vi "IP Address - Get.vi"(11 "error in (no error)":errorcluster) -> (4 "return code":i32, 6 "LAN IP Address":string, 8 "LAN Subnet Mask":string, 15 "error out":errorcluster)   [LabVIEW 2009]
panel:
  out "Wireless IP Address":string
  out "Wireless Subnet Mask":string
  out "standard output":string
  out "standard error":string
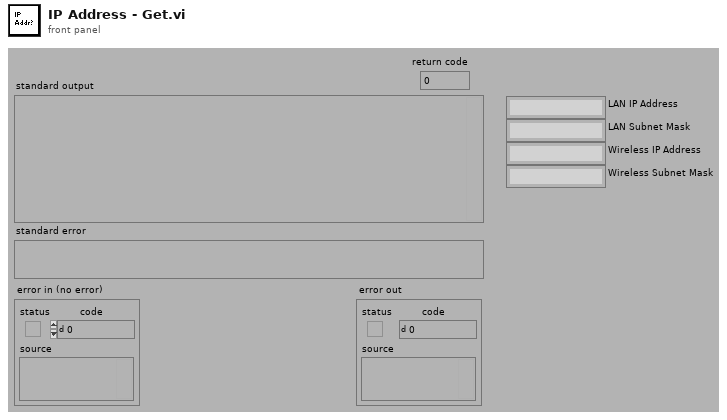
[diagram p1: front panel]
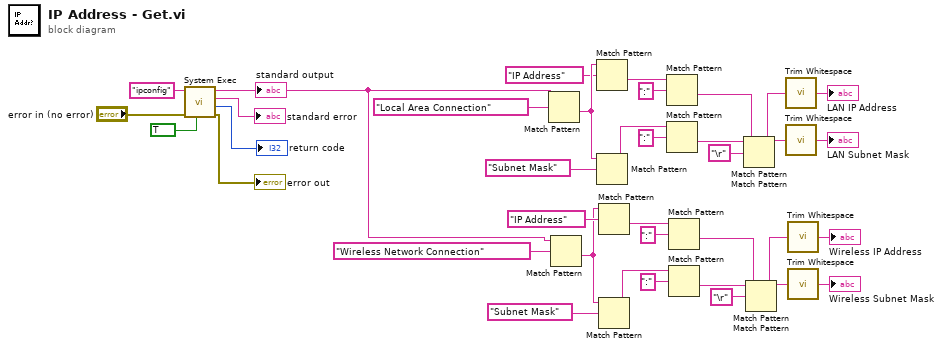
[diagram p0: block diagram]
diagram:
  n1 = call <vilib>:"System Exec.vi"("run minimized? (F)"=TRUE, "error in (no error)"="error in (no error)", "command line"="ipconfig") -> ("error out"=→"error out":errorcluster, "return code"=→"return code":i32, "standard error"=→"standard error":string, "standard output"=w1:string)  [unwired: 5 in]
  "standard output" <- w1
  n2 = Match Pattern(string=w1, regular expression="Local Area Connection" ("command line")) -> (after substring=w27:string)  [unwired: 1 in, 3 out]
  n3 = Match Pattern(string=w1, regular expression="Wireless Network Connection" ("command line")) -> (after substring=w11:string)  [unwired: 1 in, 3 out]
  n4 = Match Pattern(string=w27, regular expression="IP Address" ("command line")) -> (after substring=w35:string)  [unwired: 1 in, 3 out]
  n5 = Match Pattern(string=w27, regular expression="Subnet Mask" ("command line")) -> (after substring=w30:string)  [unwired: 1 in, 3 out]
  n6 = Match Pattern(string=w11, regular expression="IP Address" ("command line")) -> (after substring=w3:string)  [unwired: 1 in, 3 out]
  n7 = Match Pattern(string=w11, regular expression="Subnet Mask" ("command line")) -> (after substring=w8:string)  [unwired: 1 in, 3 out]
  n8 = Match Pattern(string=w35, regular expression=":" ("command line")) -> (after substring=w28:string)  [unwired: 1 in, 3 out]
  n9 = Match Pattern(string=w30, regular expression=":" ("command line")) -> (after substring=w29:string)  [unwired: 1 in, 3 out]
  n10 = Match Pattern(string=w3, regular expression=":" ("command line")) -> (after substring=w10:string)  [unwired: 1 in, 3 out]
  n11 = Match Pattern(string=w8, regular expression=":" ("command line")) -> (after substring=w9:string)  [unwired: 1 in, 3 out]
  n12 = Match Pattern(string=w29, regular expression="\r" ("command line")) -> (before substring=w23:string)  [unwired: 1 in, 3 out]
  n13 = Match Pattern(string=w28, regular expression="\r" ("command line")) -> (before substring=w21:string)  [unwired: 1 in, 3 out]
  n14 = Match Pattern(string=w9, regular expression="\r" ("command line")) -> (before substring=w15:string)  [unwired: 1 in, 3 out]
  n15 = Match Pattern(string=w10, regular expression="\r" ("command line")) -> (before substring=w17:string)  [unwired: 1 in, 3 out]
  n16 = call <vilib>:"Trim Whitespace.vi"("string"=w21) -> ("trimmed string"=→"LAN IP Address":string)  [unwired: 1 in]
  n17 = call <vilib>:"Trim Whitespace.vi"("string"=w23) -> ("trimmed string"=→"LAN Subnet Mask":string)  [unwired: 1 in]
  n18 = call <vilib>:"Trim Whitespace.vi"("string"=w17) -> ("trimmed string"=→"Wireless IP Address":string)  [unwired: 1 in]
  n19 = call <vilib>:"Trim Whitespace.vi"("string"=w15) -> ("trimmed string"=→"Wireless Subnet Mask":string)  [unwired: 1 in]
